vi "DataLog Dump Tag Buffer_srv.vi"(7 "certificate":string, 11 "tag":string) -> (8 "points":T1[](array[typedef]) {"value" format="%.3e"; "time" format="%<%H:%M:%S%2u\n%Y/%m/%d>T"}, 15 "error out":errorcluster)   [LabVIEW 2012]
doc: "Reads all (when initial is true) or newer (when initial is false) data points from the in-memory buffers of a subset of tags. The read indices beyond the last read point are also returned. This allows a remote exhaustive read of multiple tags using a single VI server call thereby minimizing network load and latency."
uses:
  typedefs/clusters/t_DataLog Point.ctl
  typedefs/t_DataLog Tag Hash Methods.ctl
  clientsrv/typedefs/t_ClientSrv Access Levels.ctl
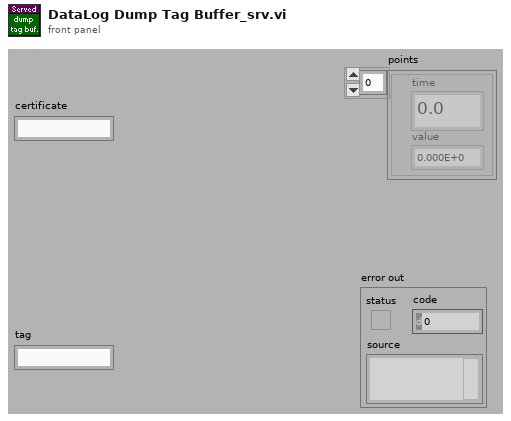
[diagram p1: front panel]
types:
  T1 = typedef "t_DataLog Point.ctl" = cluster{"time":dbl, "value":dbl}
  T2 = typedef "t_ClientSrv Access Levels.ctl" = enum16{"observer", "operator", "local"}
  T3 = typedef "t_DataLog Tag Hash Methods.ctl" = enum16{"initialize", "add tag", "index tag", "lookup", "#tags", "cleanup", "write recovery", "read recovery", "delete recovery"}
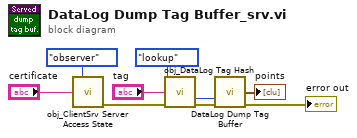
[diagram p0: block diagram]
diagram:
  n1 = call "obj_ClientSrv Server Access State.vi"("access level"=t_ClientSrv_Access_Levels."observer", "certificate in"="certificate") -> ("error out"=w7:errorcluster)  [unwired: 11 in, 2 out]
  n2 = call "obj_DataLog Tag Hash.vi"("method"=t_DataLog_Tag_Hash_Methods."lookup", "tag in"="tag", "error in (no error)"=w7) -> ("tag index out"=w3:i32, "error out"=w4:errorcluster)  [unwired: 9 in, 2 out]
  n3 = call "DataLog Dump Tag Buffer.vi"("tag index"=w3, "error in (no error)"=w4) -> ("points"=→"points":T1[], "error out"=→"error out":errorcluster)  [unwired: 10 in, 2 out]
